vi "Create IAbortHandler.vi"(8 "error in (no error)":errorcluster, 11 "IWampMessage":refnum<class "IWampMessage.lvclass">) -> (0 "error out":errorcluster, 3 "IAbortHandler":refnum<class "IAbortHandler.lvclass">)   [LabVIEW 2020, in "wamplv.lvlib"]
uses:
  wamplv.lvlib
  SerialisedMessages/JSONMessage/WampMessage JSON.lvclass
  SerialisedMessages/MsgPackMessage/WampMessage MsgPack.lvclass
  SerialisedMessages/IWampMessage/IWampMessage.lvclass
  Error/AbortHandler MsgPack/AbortHandler MsgPack.lvclass
  AbortHandler JSON/AbortHandler JSON.lvclass
  C:/local/wamplv/Private/Requests/MessageReceivedHandlers/Error/IAbortOrErroHandler/IAbortOrErrorHandler.lvclass
  C:/local/wamplv/Private/Requests/IInternalMessage/IInternalMessage.lvclass
  C:/local/wamplv/Private/Requests/MessageReceivedHandlers/Error/IAbortHandler/IAbortHandler.lvclass
  C:/local/wamplv/Private/Requests/MessageReceivedHandlers/Error/AbortHandler JSON/AbortHandler JSON.lvclass
  C:/local/wamplv/Private/Requests/MessageReceivedHandlers/IJsonMessageHandler/IJsonMessageHandler.lvclass
  C:/local/wamplv/Private/Requests/Error/AbortHandler MsgPack/AbortHandler MsgPack.lvclass
  C:/local/wamplv/Private/Requests/MessageReceivedHandlers/IMsgPackMessageHandler/IMsgPackMessageHandler.lvclass
  IAbortHandler/IAbortHandler.lvclass
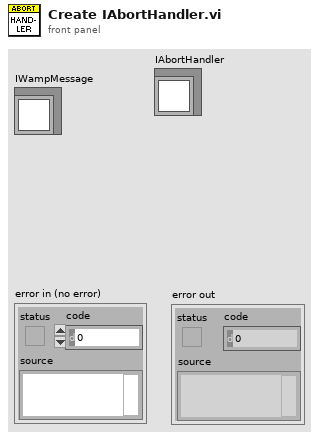
[diagram p1: front panel]
types:
  T1 = typedef "wamplv.lvlib/WAMP Client.lvclass/Serialisation.ctl" = enum16{"JSON", "MessagePack"}
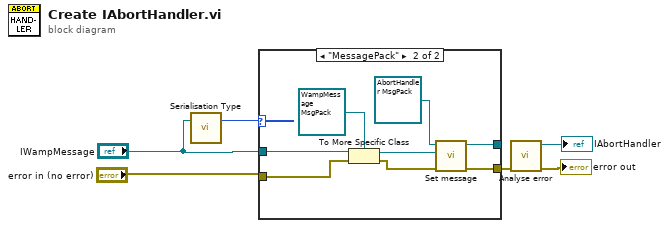
[diagram p0: block diagram]
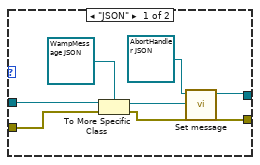
[diagram p2: hidden frame]
diagram:
  n1 = call-dynamic "Serialisation Type.vi"("IWampMessage in"="IWampMessage") -> ("Serialisation Type"=w6:T1)  [unwired: 2 in]
  n2 = case shown="\"MessagePack\"" w6 {
    tunnel: "IWampMessage" -> [w13 w20]
    tunnel: "error in (no error)" -> [w11 w19]
    tunnel: [w7 w17] -> w3
    tunnel: [w9 w14] -> _
    frame "JSON" {
      n3 = To More Specific Class(target class=refnum<class "WampMessage JSON.lvclass"> refnum ("wamplv.lvlib:JSONMessage.lvclass"), reference=w13, error in=w11) -> (specific class reference=w10:refnum<class "WampMessage JSON.lvclass">, error out=w7:errorcluster)
      n4 = call-dynamic "Set message.vi"("WampMessage JSON"=w10, "AbortHandler JSON in"=refnum<class "AbortHandler JSON.lvclass"> refnum ("wamplv.lvlib:AbortHandler JSON.lvclass")) -> ("AbortHandler JSON out"=w9:refnum<class "AbortHandler JSON.lvclass">)  [unwired: 9 in]
    }
    frame "MessagePack" {
      n5 = To More Specific Class(target class=refnum<class "WampMessage MsgPack.lvclass"> refnum ("wamplv.lvlib:MsgPackMessage.lvclass"), reference=w20, error in=w19) -> (specific class reference=w15:refnum<class "WampMessage MsgPack.lvclass">, error out=w17:errorcluster)
      n6 = call-dynamic "Set message.vi"("WampMessage MsgPack"=w15, "AbortHandler MsgPack in"=refnum<class "AbortHandler MsgPack.lvclass"> refnum ("wamplv.lvlib:AbortHandler MsgPack.lvclass")) -> ("AbortHandler MsgPack out"=w14:refnum<class "AbortHandler MsgPack.lvclass">)  [unwired: 9 in]
    }
  }
  n7 = call-dynamic "Analyse error.vi"("error in (no error)"=w3) -> ("error out"=→"error out":errorcluster, "IErrorHandler out"=→"IAbortHandler":refnum<class "AbortHandler JSON.lvclass">)  [unwired: 9 in]
